vi "SetStagePixel.vi"(9 "Scan Mode":enum16{"Raster Scan", "Serpentine Scan"}(ring), 10 "Line Count":i32, 11 "Pixel Count":i32) -> (1 "Y Pixel":i32, 2 "X Pixel":i32, 3 "Completed?":bool)   [LabVIEW 2018]
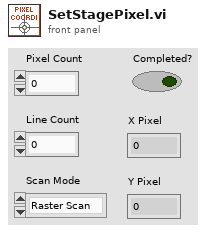
[diagram p1: front panel]
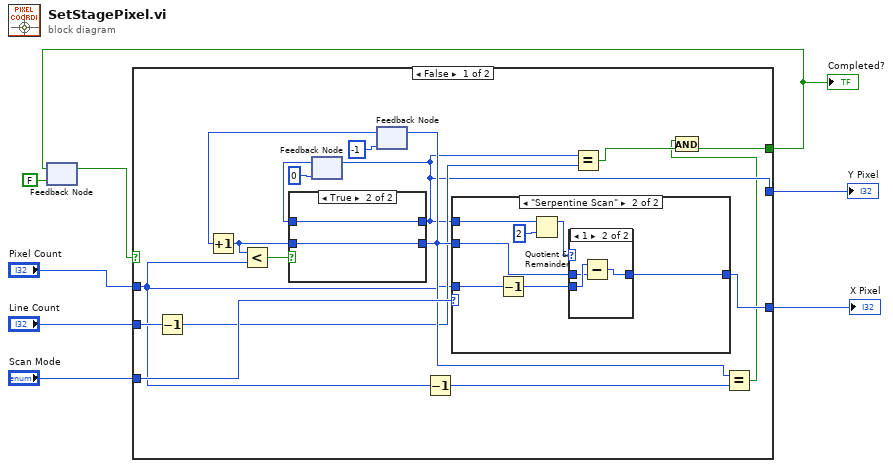
[diagram p0: block diagram]
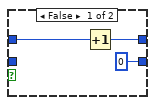
[diagram p4: hidden frame]
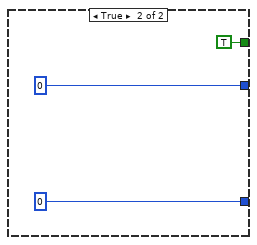
[diagram p5: hidden frame]
diagram:
  n1 = feedback #1(FALSE) -> (w3:bool)
  n2 = case shown="False" w3 {
    tunnel: "Line Count" -> [w25 _]
    tunnel: "Pixel Count" -> [w10 _]
    tunnel: "Scan Mode" -> [w24 _]
    tunnel: [w14 0] -> w5
    tunnel: [w12 TRUE] -> w2
    tunnel: [w13 0] -> w4
    frame False {
      n3 = Decrement(x=w25) -> (x-1=w15:i32)
      n4 = feedback #2(0) -> (w20:i32)
      n5 = feedback #3(-1) -> (w16:i32)
      n6 = Increment(x=w16) -> (x+1=w18:i32)
      n7 = Less?(x=w18, y=w10) -> (x < y?=w17:bool)
      n8 = case shown="True" w17 {
        tunnel: w18 -> [_ w42]
        tunnel: [0 w42] -> w19
        tunnel: w20 -> [w39 w41]
        tunnel: [w38 w41] -> w14
        frame False {
          n9 = Increment(x=w39) -> (x+1=w38:i32)
        }
        frame True {
        }
      }
      n10 = feedback-in #2(w14) -> ()
      n11 = feedback-in #3(w19) -> ()
      n12 = Decrement(x=w10) -> (x-1=w9:i32)
      n13 = case shown="\"Serpentine Scan\"" w24 {
        tunnel: w14 -> [_ w31]
        tunnel: w10 -> [_ w28]
        tunnel: w19 -> [w26 w30]
        tunnel: [w26 w29] -> w13
        frame "Raster Scan", Default {
        }
        frame "Serpentine Scan" {
          n14 = Decrement(x=w28) -> (x-1=w27:i32)
          n15 = Quotient & Remainder(x=w31, y=2) -> (x-y*floor(x/y)=w32:i32)  [unwired: 1 out]
          n16 = case shown="1" w32 {
            tunnel: w30 -> [w34 w36]
            tunnel: [w34 w35] -> w29
            tunnel: w27 -> [_ w37]
            frame 0, Default {
            }
            frame 1 {
              n17 = Subtract(x=w37, y=w36) -> (x-y=w35:i32)
            }
          }
        }
      }
      n18 = Equal?(x=w14, y=w15) -> (x = y?=w21:bool)
      n19 = Equal?(x=w19, y=w9) -> (x = y?=w11:bool)
      n20 = And(x=w11, y=w21) -> (x .and. y?=w12:bool)
    }
    frame True {
    }
  }
  "Y Pixel" <- w5
  "Completed?" <- w2
  "X Pixel" <- w4
  n21 = feedback-in #1(w2) -> ()
